vi "formatAttributeString.vi"(8 "error in (no error)":errorcluster, 10 "attributeElement":T1, 11 "WriteAttribute in":refnum<class "XMLAttributeGenerator.lvclass">) -> (0 "error out":errorcluster, 2 "String":string, 3 "WriteAttribute out":refnum<class "XMLAttributeGenerator.lvclass">)   [LabVIEW 2016, in "XML.lvlib" / "XMLAttributeGenerator.lvclass"]
doc: "This method simply takes the attribute element and formats it into the form AttributeType=\"AttributeValue\""
uses:
  <userlib>/Common/XML/XMLAttributeGenerator/XMLAttributeGenerator.lvclass
  <userlib>/Common/XML/Typedefs/AttributeElements.ctl
  <userlib>/Common/XML/XML.lvlib
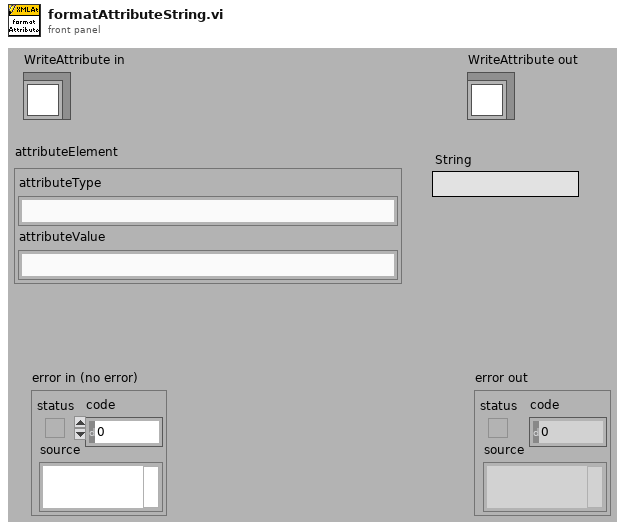
[diagram p1: front panel]
types:
  T1 = typedef "XML.lvlib/AttributeElements.ctl" = cluster{"attributeType":string, "attributeValue":string}
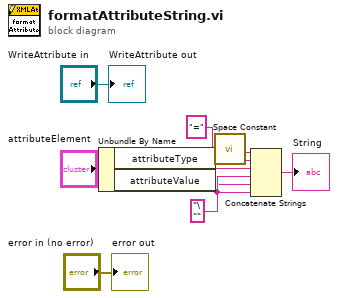
[diagram p0: block diagram]
diagram:
  w6 = "\"" ("string")
  n1 = Unbundle By Name("attributeElement") -> ("attributeType"=w3:string, "attributeValue"=w5:string)
  n2 = call <vilib>:"Space Constant.vi"() -> ("String"=w7:string)
  n3 = Concatenate Strings(w7, w3, "=" ("string"), w6, w5, w6) -> (→"String":string)
  "WriteAttribute out" <- "WriteAttribute in"
  "error out" <- "error in (no error)"
